vi "Msg.vi"(7 "LVCAM in":refnum<class "LVCAM.lvclass">, 11 "Open UI Msg in":refnum<class "Open UI Msg.lvclass">) -> (0 "error out":errorcluster, 5 "LVCAM out":refnum<class "LVCAM.lvclass">)   [LabVIEW 2021, in "Open UI.lvlib" / "Open UI Msg.lvclass"]
uses:
  Open UI Msg.lvclass
  LVCAM/LVCAM/LVCAM/LVCAM.lvclass
  Open UI/Open UI.lvclass
  3a537078-b41c-4e7b-bfaf-9491628aff3f.vi
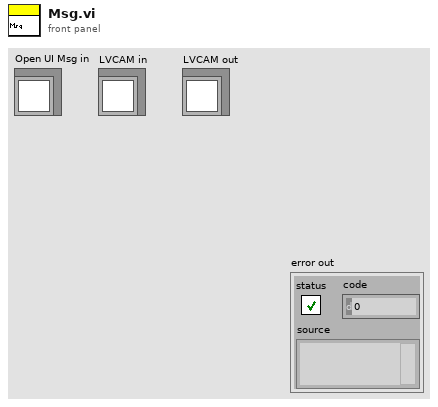
[diagram p1: front panel]
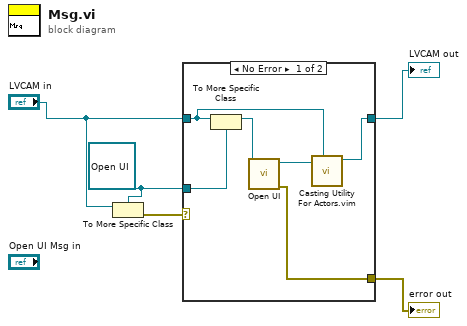
[diagram p0: block diagram]
diagram:
  w1 = refnum<class "Open UI.lvclass"> refnum ("Open UI.lvlib:Open UI.lvclass")
  n1 = To More Specific Class(target class=w1, reference="LVCAM in") -> (error out=w5:errorcluster)  [unwired: 1 in, 1 out]
  n2 = case shown="No Error" w5 {
    selector: w5 -> [_ w13]
    tunnel: [w9 w13] -> w4
    tunnel: [w6 w12] -> w3
    tunnel: "LVCAM in" -> [w7 w12]
    tunnel: w1 -> [w11 _]
    frame No Error {
      n3 = To More Specific Class(target class=w11, reference=w7) -> (specific class reference=w10:refnum<class "Open UI.lvclass">)  [unwired: 1 in, 1 out]
      n4 = call-dynamic "Open UI.vi"("Open UI in"=w10) -> ("error out"=w9:errorcluster, "Open UI out"=w8:refnum<class "Open UI.lvclass">)  [unwired: 9 in]
      n5 = call "Casting Utility For Actors.vim"("type"=w7, "Actor in"=w8) -> ("Actor out"=w6:refnum<class "LVCAM.lvclass">)  [unwired: 8 in, 1 out]
    }
    frame Error {
    }
  }
  "error out" <- w4
  "LVCAM out" <- w3
